vi "onAssertionSlippage.vi"(7 "RequirementsFile in":refnum<class "RequirementMap.lvclass">, 11 "Leaf.Assertion":refnum<class "Leaf.Assertion.lvclass">) -> (0 "error out":errorcluster, 3 "Leaf.Assertion":refnum<class "Leaf.Assertion.lvclass">)   [LabVIEW 2021, in "Bananas.lvlib" / "RequirementMap.lvclass"]
uses:
  RequirementMap.lvclass
  RequirementMap.lvclass/RequirementMap.ctl
  Leaf.Assertion/Leaf.Assertion.lvclass
  C:/Repositories/LVOS/Bananas/lv-src/Bananas/Leaf.Assertion/Leaf.Assertion.lvclass
  C:/Repositories/LVOS/Bananas/lv-src/Bananas/Leaf/Leaf.lvclass
  Leaf/Leaf.lvclass
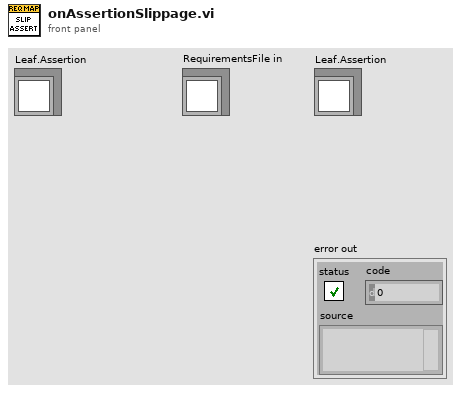
[diagram p1: front panel]
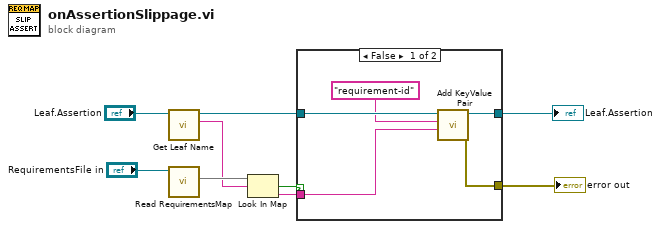
[diagram p0: block diagram]
diagram:
  n1 = call "Get Leaf Name.vi"("Leaf in"="Leaf.Assertion") -> ("Name"=w2:string, "Leaf out"=w1:refnum<class "Leaf.Assertion.lvclass">)  [unwired: 8 in, 1 out]
  n2 = call "Read RequirementsMap.vi"("RequirementsFile in"="RequirementsFile in") -> ("Requirements"=w8:map{string, string})  [unwired: 9 in, 1 out]
  n3 = Look In Map(map=w8, key=w2) -> (key not found?=w7:bool, value=w5:string)  [unwired: 1 in]
  n4 = case shown="False" w7 {
    tunnel: [w11 w15] -> w6
    tunnel: w1 -> [w14 w15]
    tunnel: w5 -> [w12 _]
    tunnel: [w10 _] -> w4
    frame False {
      n5 = call "Add KeyValue Pair.vi"("value"=w12, "key"="requirement-id", "Leaf in"=w14) -> ("error out"=w10:errorcluster, "Leaf out"=w11:refnum<class "Leaf.Assertion.lvclass">)  [unwired: 7 in]
    }
    frame True {
    }
  }
  "error out" <- w4
  "Leaf.Assertion" <- w6
